vi "Start Command.vi"(8 "error in":errorcluster, 11 "CoreOOB_Rx in":refnum<class "CIFCoreOOB_Rx.lvclass">) -> (0 "error out":errorcluster, 3 "CoreOOB_Rx out":refnum<class "CIFCoreOOB_Rx.lvclass">)   [LabVIEW 2021, in "CIFCoreOOB_Rx.lvclass"]
uses:
  CIFCoreOOB_Rx.lvclass
  D:/dev/CIF-LVCore/src/CIFUtilities/CIFOutOfBand/CIFOutOfBand.lvclass
  Typedef/OOB Core Commands.ctl
  CIFUtilities/CIFOutOfBand/CIFOutOfBand.lvclass/CIFOutOfBand.ctl
  CIFCoreOOB_Rx.lvclass/CIFCoreOOB_Rx.ctl
  CIFUtilities/CIFOutOfBand/CIFOutOfBand.lvclass
  D:/dev/CIF-LVCore/src/CIFCore/OOB/OOB_Rx/CIFCoreOOB_Rx.lvclass
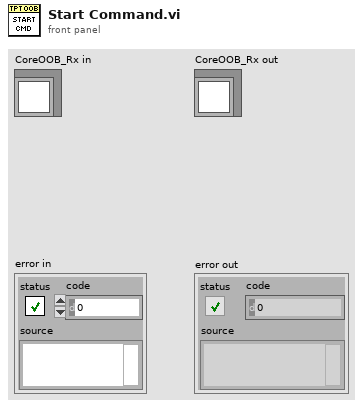
[diagram p1: front panel]
types:
  T1 = typedef "CIFCoreOOB_Rx.lvclass/OOB Core Commands.ctl" = enum8{"Start", "Pause", "Stop", "RefreshStats", "UpdateConfig"}
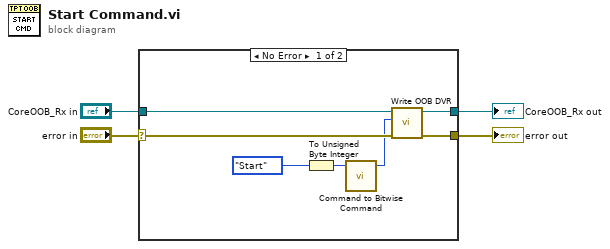
[diagram p0: block diagram]
diagram:
  n1 = case shown="No Error" "error in" {
    selector: "error in" -> [w9 w13]
    tunnel: [w10 w13] -> w3
    tunnel: "CoreOOB_Rx in" -> [w8 w12]
    tunnel: [w11 w12] -> w1
    frame No Error {
      n2 = To Unsigned Byte Integer(number=OOB_Core_Commands."Start" ("OOB Main Commands")) -> (unsigned 8bit integer=w7:u8)
      n3 = call "Command to Bitwise Command.vi"("OOB Command"=w7) -> ("bit command"=w6:u64)  [unwired: 3 in]
      n4 = call "Write OOB DVR.vi"("error in"=w9, "Commands (bitwise)"=w6, "OOB in"=w8) -> ("error out"=w10:errorcluster, "OOB out"=w11:refnum<class "CIFCoreOOB_Rx.lvclass">)  [unwired: 7 in]
    }
    frame Error {
    }
  }
  "error out" <- w3
  "CoreOOB_Rx out" <- w1
